vi "Live_Example.vi"() -> ()   [LabVIEW 2026]
doc: "This example demonstrates the image acquisition with one camera in ring buffer mode together with a live display of the latest images during record. After record is stopped, the images can be addressed by index.\nNote that this example will not be fail save, i.e. doesnt react on errors, just handles them forward to the end\n\nUsage:\nSelect your required image count, data format and the camera setup before you start the program.\nOnce started, the camera class will be initialized and images will be recorded and displayed automatically\nYou can stop the images by pressing stop record.\nAfter stopped, the image at the selected index will be read out\nTo finish the program click on quit application, this will force an exit of the camera class\nYou can change your required ROI after and also during the record."
uses:
  <instrlib>/PCO_SDK/File Group 0/vi.lib/Excelitas PCO GmbH/pco.labview/camera/Camera.lvclass
  <vilib>/picture/picture.llb/Draw 8-Bit Pixmap.vi
  <vilib>/picture/picture.llb/Draw True-Color Pixmap.vi
  <instrlib>/PCO_SDK/File Group 0/vi.lib/Excelitas PCO GmbH/pco.labview/pco.sdk/TimingControl/TimingControl.lvlib
panel:
  out "colormap(U8)":u32[](array[numeric])
  in  "Zoom [%]":i32(slide)=26 min=10 max=200 step=5 scale=10.0..200.0
  out "Image":picture
  out "Image(U16)":u16[][](graph)
  in  "Trigger":bool
  in  "data_format":T1(ring)=enum."Mono16"
  out "rawImage":u16[][](array[numeric])
  in  "Image Index":u32
  out "Recorded Images":u32
  in  "TriggerMode":T2(ring)
  in  "Quit":bool
  out "Error":errorcluster {"code" format="%x"}
  in  "Stop Record":bool
  out "Recording On":bool
  in  "roiY1":u64=2 min=1 max=1 step=1
  in  "roiX1":u64=2 min=1 max=1 step=1
  in  "roiY0":u64=1 max=1 step=1
  in  "roiX0":u64=1 max=1 step=1
  out "Image Height":u64
  out "Image Width":u64
  in  "dwImgCount":u32=10 caption="Required Number of Images" max=2397
  in  "Exposure Time [s]":dbl=0.010000000000000002 step=0.001
  # "This example demonstrates the image acquisition with one camera in ring buffer mode together with a live display of the latest images during record. After record is stopped, the images can be addressed by index.\nNote that this example will not be fail save, i.e. doesnt react on errors, just handles them forward to the end\n\nUsage:\nSelect your required image count, data format and the camera setup before you start the program.\nOnce started, the camera class will be initialized and images will be recorded and displayed automatically\nYou can stop the images by pressing stop record.\nAfter stopped, the image at the selected index will be read out\nTo finish the program click on quit application, this will force an exit of the camera class\nYou can change your required ROI after and also during the record."
  # "pco.labview"
  # "Camera Setup"
  # "Recording Control"
  # "Parameters for image readout"
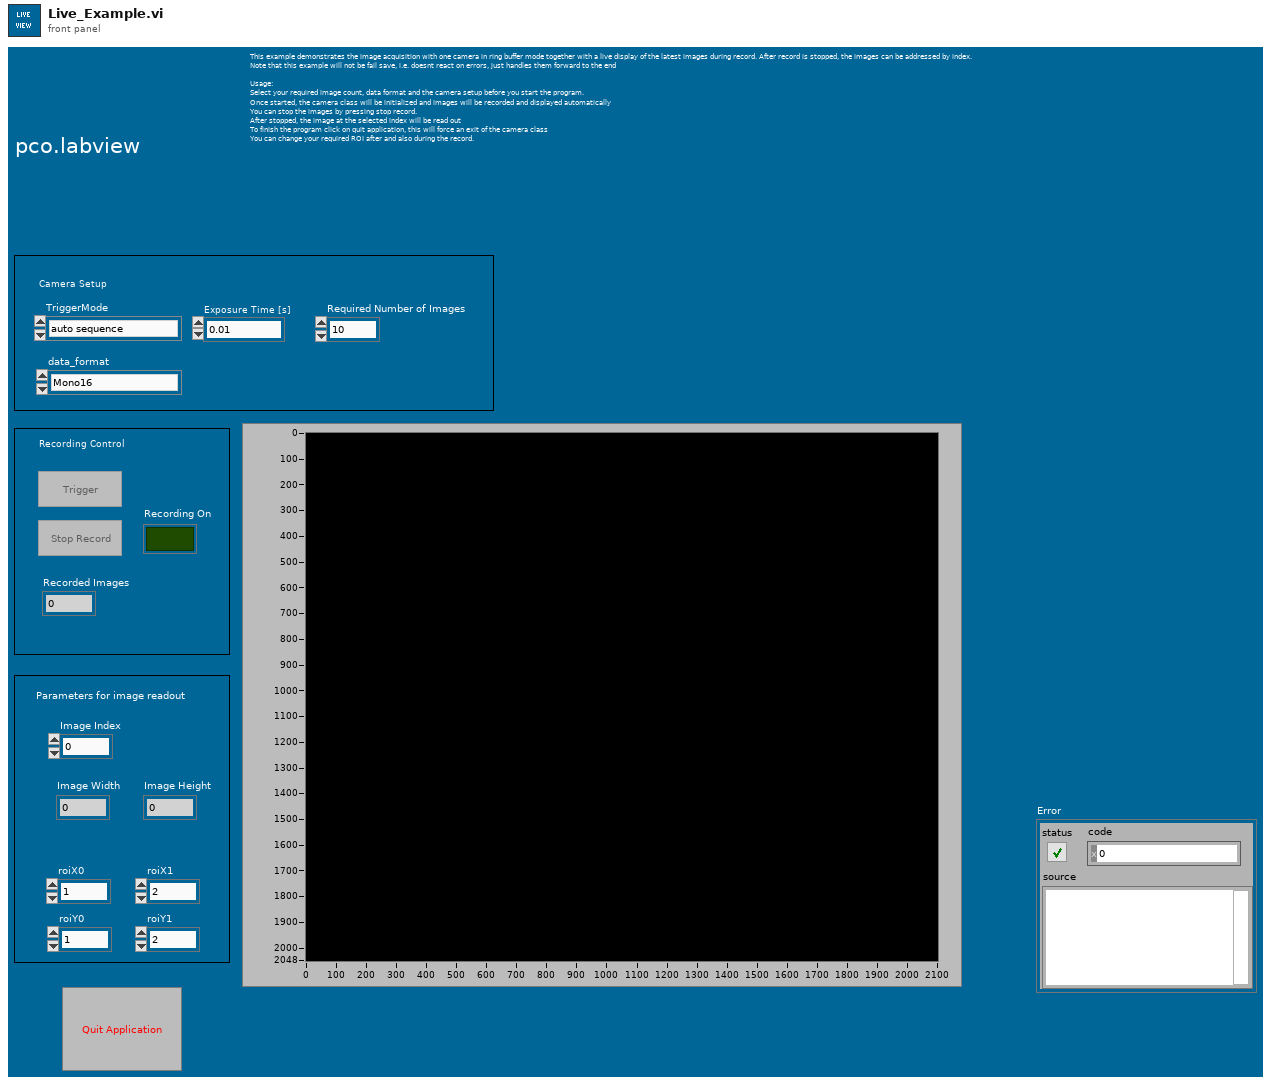
[diagram p1: front panel]
types:
  T1 = enum16{"Undefined", "Mono8", "Mono16", "BGRA8", "RGBA8", "BGRA16", "RGBA16", "CompressedMono8"}
  T2 = enum16{"auto sequence", "software trigger", "external exposure start", "external exposure control"}
  T3 = enum16{"sequence", "sequence non blocking", "ring buffer", "fifo", "sequence_dpcore", "sequence_non_blocking_dpcore", "ring_buffer_dpcore", "fifo_dpcore", "tif", "multitif", "pcoraw", "b16", "dicom", "multidicom", "camram_ring", "camram_segment"}
  T4 = enum8{"Enabled", "Disabled", "Disabled and Grayed Out"}
  T5 = cluster{"serial":u32, "type":u16, "sub_type":u16, "interface_type":u16, "bit_resolution":u16, "min_exposure_time_s":dbl, "max_exposure_time_s":dbl, "min_exposure_step_s":dbl, "min_delay_time_s":dbl, "max_delay_time_s":dbl, "min_delay_step_s":dbl, "min_width":u64, "min_height":u64, "max_width":u64, "max_height":u64, "roi_step_horz":u64, "roi_step_vert":u64, "roi_symmetric_horz":bool, "roi_symmetric_vert":bool, "has_timestamp_mode":bool, "has_timestamp_mode_ascii_only":bool, "pixelrate_vec":u32[], "has_acquire_mode":bool, "has_ext_acquire_mode":bool, "has_metadata_mode":bool, "has_ram":bool, "binning_horz_vec":u16[], "binning_vert_vec":u16[], "has_average_binning":bool, "pixel_format_vec":u32[], "has_trigger_mode_extexpctrl":bool}
  T6 = cluster{"wSignalNum":u16, "wEnabled":u16, "wType":u16, "wPolarity":u16, "wFilterSetting":u16, "wSelected":u16, "dwParameter":u32[], "dwSignalFunctionality":u32[]}
  T7 = typedef "Camera.lvclass/binning.ctl" = cluster{"vert":u16, "horz":u16, "mode":u16}
  T8 = cluster{"exposure_time_s":dbl, "delay_time_s":dbl, "roi":cluster{"x0":u64, "y0":u64, "x1":u64, "y1":u64}, "timestamp_mode":u16, "pixelrate":u32, "trigger_mode":u16, "acquire_mode":u16, "metadata_mode":u16, "noisefilter_mode":u16, "pixel_format":u32, "binning":T7, "auto_exposure":cluster{"region":u16, "min_exposure_s":dbl, "max_exposure_s":dbl}}
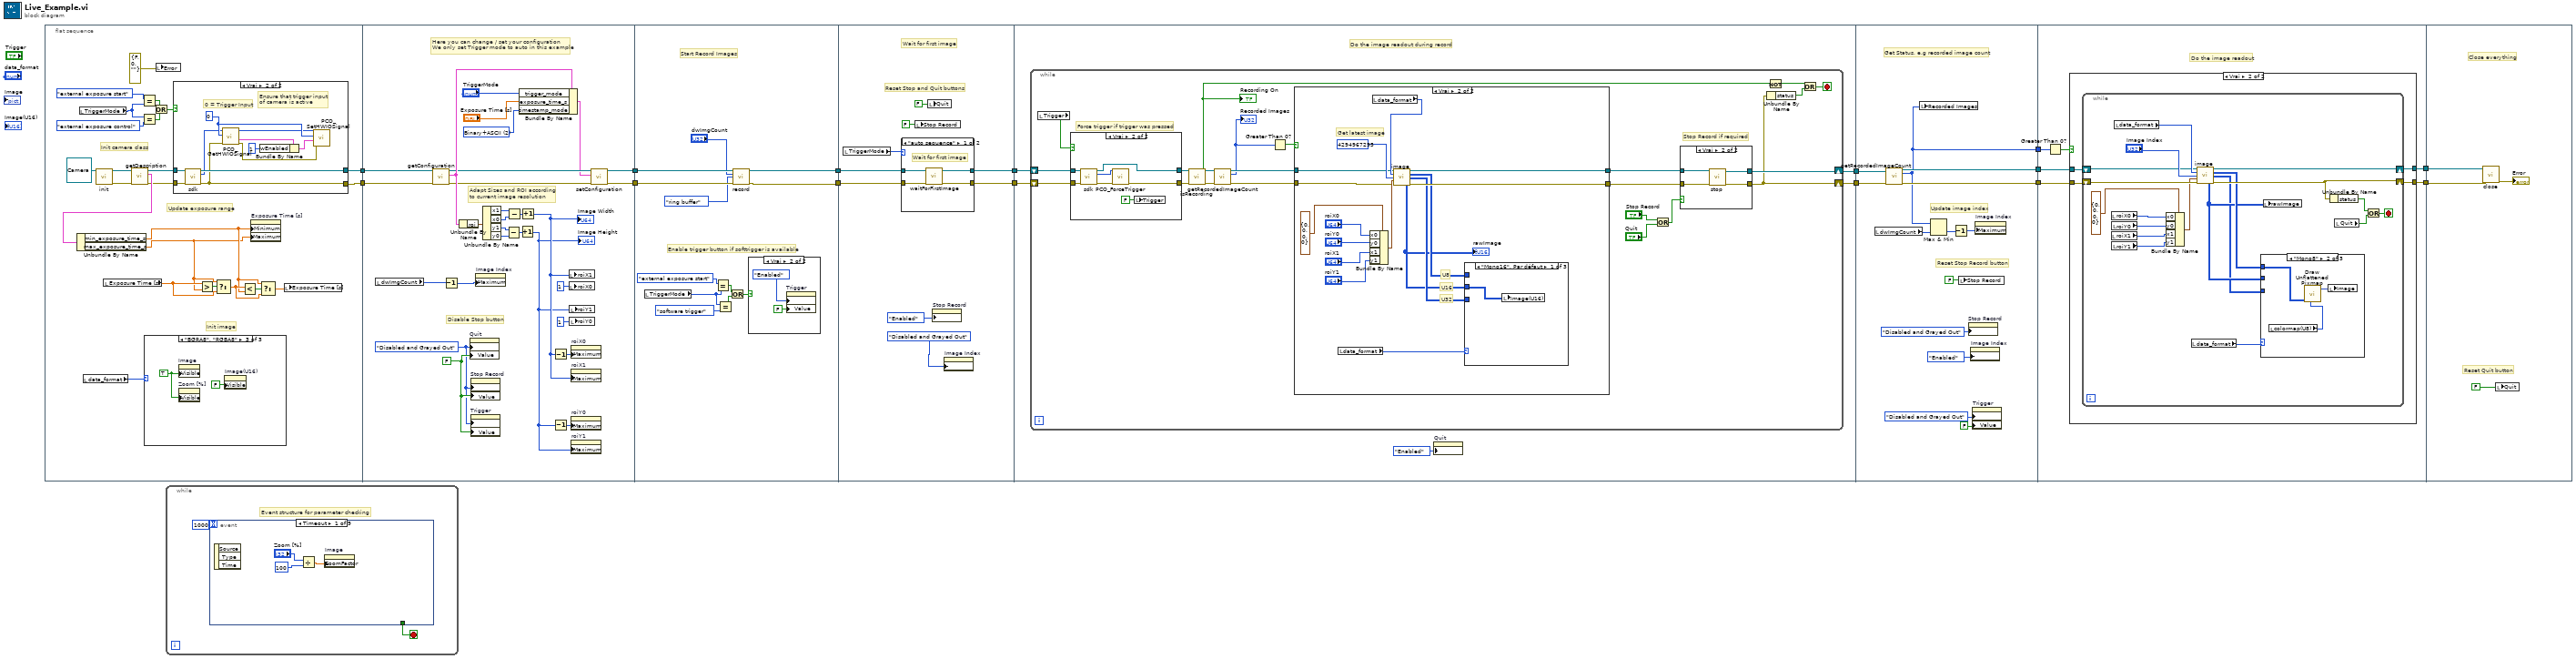
[diagram p0: block diagram]
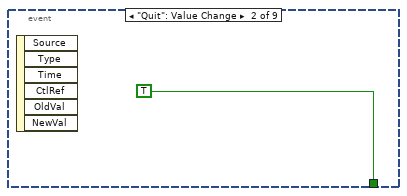
[diagram p2: hidden frame]
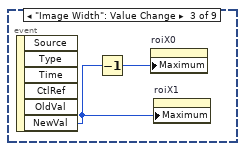
[diagram p3: hidden frame]
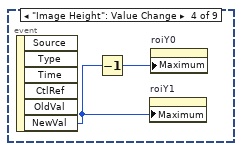
[diagram p4: hidden frame]
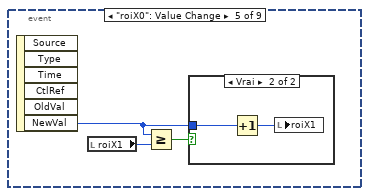
[diagram p5: hidden frame]
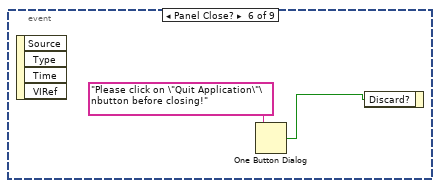
[diagram p7: hidden frame]
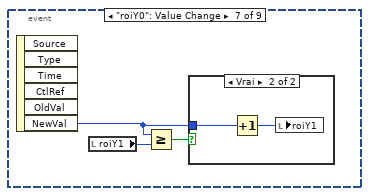
[diagram p8: hidden frame]
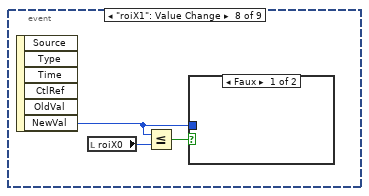
[diagram p10: hidden frame]
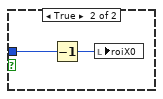
[diagram p11: hidden frame]
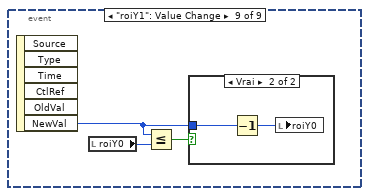
[diagram p12: hidden frame]
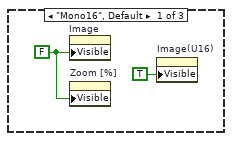
[diagram p15: hidden frame]
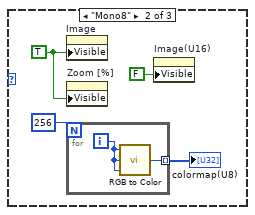
[diagram p16: hidden frame]
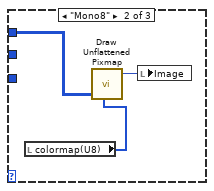
[diagram p20: hidden frame]
diagram:
  n1 = flat-sequence {
    tunnel: [w23] -> w7
    tunnel: [w16] -> w6
    tunnel: [w66] -> w15
    tunnel: [w70] -> w14
    tunnel: w7 -> [w65]
    tunnel: w6 -> [w64]
    tunnel: [w91] -> w9
    tunnel: [w92] -> w8
    tunnel: w14 -> [w101]
    tunnel: w15 -> [w100]
    tunnel: w9 -> [w108]
    tunnel: w8 -> [w109]
    tunnel: [w107] -> w13
    tunnel: [w105] -> w2
    tunnel: w13 -> [w123]
    tunnel: [w121] -> w12
    tunnel: [w120] -> w5
    tunnel: w2 -> [w119]
    tunnel: w12 -> [w194]
    tunnel: [w192] -> w11
    tunnel: w5 -> [w187]
    tunnel: [w186] -> w4
    tunnel: [w185] -> w1
    tunnel: w11 -> [w203]
    tunnel: [w202] -> w10
    tunnel: w4 -> [w201]
    tunnel: [w200] -> w3
    tunnel: w1 -> [w198]
    tunnel: w10 -> [w237]
    tunnel: w3 -> [w235]
    frame #0 {
      # "Init image"
      # "Init camera class"
      # "Update exposure range"
      n2 = local read "TriggerMode"() -> (w21:T2)
      n3 = local read "data_format"() -> (w26:T1)
      n4 = call-dynamic "init.vi"("Camera in"=refnum<class "Camera.lvclass"> refnum) -> ("Camera out"=w30:refnum<class "Camera.lvclass">, "error out"=w31:errorcluster)  [unwired: 8 in]
      n5 = local read "Exposure Time [s]"() -> (w37:dbl)
      n6 = call-dynamic "getDescription.vi"("error in (no error)"=w31, "Camera in"=w30) -> ("error out"=w25:errorcluster, "description"=w29:T5, "Camera out"=w24:refnum<class "Camera.lvclass">)  [unwired: 7 in]
      n7 = Unbundle By Name(w29) -> ("min_exposure_time_s"=w28:dbl, "max_exposure_time_s"=w27:dbl)
      n8 = Equal?(x=T2."external exposure start" ("TriggerMode"), y=w21) -> (x = y?=w19:bool)
      n9 = Equal?(x=w21, y=T2."external exposure control" ("TriggerMode")) -> (x = y?=w18:bool)
      n10 = case shown="\"BGRA8\", \"RGBA8\"" w26 {
        frame "Mono16", Default {
          w52 = FALSE ("Visible")
          n11 = property on="Image" class="Image"("Visible"=w52) -> ()  [unwired: 2 in, 2 out]
          n12 = property on="Zoom [%]" class="Gliss (strict)"("Visible"=w52) -> ()  [unwired: 2 in, 2 out]
          n13 = property on="Image(U16)" class="GraphInt (strict)"("Visible"=TRUE) -> ()  [unwired: 2 in, 2 out]
        }
        frame "Mono8" {
          w56 = TRUE ("Visible")
          n14 = property on="Image" class="Image"("Visible"=w56) -> ()  [unwired: 2 in, 2 out]
          n15 = property on="Zoom [%]" class="Gliss (strict)"("Visible"=w56) -> ()  [unwired: 2 in, 2 out]
          n16 = for {
            N: 256 -> [_]
            tunnel: [w58] -> w55 mode=indexing
            i -> [w59]
            n17 = call <vilib>:"RGB to Color.vi"("B"=w59, "G"=w59, "R"=w59) -> ("Color"=w58:u32)
          }
          "colormap(U8)" <- w55
          n18 = property on="Image(U16)" class="GraphInt (strict)"("Visible"=FALSE) -> ()  [unwired: 2 in, 2 out]
        }
        frame "BGRA8", "RGBA8" {
          w60 = TRUE ("Visible")
          n19 = property on="Image" class="Image"("Visible"=w60) -> ()  [unwired: 2 in, 2 out]
          n20 = property on="Zoom [%]" class="Gliss (strict)"("Visible"=w60) -> ()  [unwired: 2 in, 2 out]
          n21 = property on="Image(U16)" class="GraphInt (strict)"("Visible"=FALSE) -> ()  [unwired: 2 in, 2 out]
        }
      }
      n22 = Or(x=w19, y=w18) -> (x .or. y?=w17:bool)
      n23 = local write "Error"(errorcluster {"status"=FALSE, "code"=0, "source"=""} ("error IO")) -> ()
      n24 = case shown="Vrai" w17 {
        tunnel: w25 -> [w39 w45]
        tunnel: w24 -> [w40 w44]
        tunnel: [w40 w43] -> w23
        tunnel: [w39 w41] -> w16
        frame False {
        }
        frame True {
          w49 = u16 0 ("wSignalNum")
          # "0 = Trigger Input"
          # "Ensure that trigger input\nof camera is active"
          n25 = call-dynamic "sdk.vi"("Camera in"=w44, "error in (no error)"=w45) -> ("Camera out"=w43:refnum<class "Camera.lvclass">, "sdk"=w42:u64, "error out"=w41:errorcluster)  [unwired: 11 in]
          n26 = call <instrlib>:"PCO_GetHWIOSignal.vi"("error in (no error)"=w41, "wSignalNum"=w49, "ph"=w42) -> ("error out"=w47:errorcluster, "strSignal"=w51:T6, "ph out"=w46:u64)  [unwired: 5 in, 1 out]
          n27 = Bundle By Name(cluster=w51, "wEnabled"=u16 1) -> (w48:T6)
          n28 = call <instrlib>:"PCO_SetHWIOSignal.vi"("error in (no error)"=w47, "strSignal"=w48, "wSignalNum"=w49, "ph"=w46) -> ()  [unwired: 5 in, 3 out]
        }
      }
      n29 = Greater?(x=w37, y=w27) -> (0:w38:bool)
      n30 = Select(t=w27, s=w38, f=w37) -> (s? t:f=w35:dbl)
      n31 = Less?(x=w35, y=w28) -> (x < y?=w36:bool)
      n32 = property on="Exposure Time [s]" class="NumNb (strict)"("Minimum"=w28, "Maximum"=w27) -> ()  [unwired: 2 in, 2 out]
      n33 = Select(t=w28, s=w36, f=w35) -> (s? t:f=w34:dbl)
      n34 = local write "Exposure Time [s]"(w34) -> ()
    }
    frame #1 {
      w76 = u16 2 items=["OFF", "Binary", "Binary+ASCII", "ASCII"] ("wTimeStampMode")
      w63 = FALSE ("Stop")
      w62 = T4."Disabled and Grayed Out" ("Disabled")
      # "Disable Stop button"
      # "Adapt Sizes and ROI according\nto current image resolution"
      # "Here you can change / set your configuration\nWe only set Trigger mode to auto in this example"
      n35 = local read "dwImgCount"() -> (w77:u32)
      n36 = call-dynamic "getConfiguration.vi"("error in (no error)"=w64, "Camera in"=w65) -> ("error out"=w71:errorcluster, "configuration"=w82:T8, "Camera out"=w73:refnum<class "Camera.lvclass">)  [unwired: 7 in]
      n37 = Decrement(x=w77) -> (x-1=w67:u32)
      n38 = Unbundle By Name(w82) -> ("roi"=w83:cluster{"x0":u64, "y0":u64, "x1":u64, "y1":u64})
      n39 = property on="Quit" class="Bool (strict)"("DisabledEnum"=w62, "Value"=w63) -> ()  [unwired: 2 in, 2 out]
      n40 = property on="Stop Record" class="Bool (strict)"("DisabledEnum"=w62, "Value"=w63) -> ()  [unwired: 2 in, 2 out]
      n41 = property on="Trigger" class="Bool (strict)"("DisabledEnum"=w62, "Value"=w63) -> ()  [unwired: 2 in, 2 out]
      n42 = property on="Image Index" class="NumNb (strict)"("Maximum"=w67) -> ()  [unwired: 2 in, 2 out]
      n43 = Unbundle By Name(w83) -> ("x1"=w85:u64, "x0"=w84:u64, "y1"=w87:u64, "y0"=w86:u64)
      n44 = Subtract(x=w87, y=w86) -> (x-y=w89:u64)
      n45 = Subtract(x=w85, y=w84) -> (x-y=w88:u64)
      n46 = Bundle By Name(cluster=w82, "trigger_mode"="TriggerMode", "exposure_time_s"="Exposure Time [s]", "timestamp_mode"=w76) -> (w72:T8)
      n47 = Increment(x=w89) -> (x+1=w68:u64)
      "Image Height" <- w68
      n48 = Increment(x=w88) -> (x+1=w69:u64)
      "Image Width" <- w69
      n49 = Decrement(x=w69) -> (x-1=w80:u64)
      n50 = Decrement(x=w68) -> (x-1=w81:u64)
      n51 = local write "roiX1"(w69) -> ()
      n52 = local write "roiX0"(u64 1 ("roiY0")) -> ()
      n53 = local write "roiY1"(w68) -> ()
      n54 = local write "roiY0"(u64 1 ("roiY0")) -> ()
      n55 = property on="roiX0" class="NumNb (strict)"("Maximum"=w80) -> ()  [unwired: 2 in, 2 out]
      n56 = property on="roiX1" class="NumNb (strict)"("Maximum"=w69) -> ()  [unwired: 2 in, 2 out]
      n57 = property on="roiY0" class="NumNb (strict)"("Maximum"=w81) -> ()  [unwired: 2 in, 2 out]
      n58 = property on="roiY1" class="NumNb (strict)"("Maximum"=w68) -> ()  [unwired: 2 in, 2 out]
      n59 = call-dynamic "setConfiguration.vi"("error in (no error)"=w71, "configuration"=w72, "Camera in"=w73) -> ("error out"=w70:errorcluster, "Camera out"=w66:refnum<class "Camera.lvclass">)  [unwired: 7 in]
    }
    frame #2 {
      # "Enable trigger button if softtrigger is available"
      # "Start Record Images"
      n60 = local read "TriggerMode"() -> (w97:T2)
      n61 = Equal?(x=T2."external exposure start" ("TriggerMode"), y=w97) -> (x = y?=w94:bool)
      n62 = Equal?(x=w97, y=T2."software trigger" ("TriggerMode")) -> (x = y?=w93:bool)
      n63 = Or(x=w94, y=w93) -> (x .or. y?=w95:bool)
      n64 = call-dynamic "record.vi"("Camera in"=w100, "num_images"="dwImgCount", "record_mode"=T3."ring buffer", "error in (no error)"=w101) -> ("Camera out"=w92:refnum<class "Camera.lvclass">, "error out"=w91:errorcluster)  [unwired: 10 in]
      n65 = case shown="Vrai" w95 {
        frame False {
        }
        frame True {
          n66 = property on="Trigger" class="Bool (strict)"("DisabledEnum"=T4."Enabled" ("Disabled"), "Value"=FALSE ("Trigger")) -> ()  [unwired: 2 in, 2 out]
        }
      }
    }
    frame #3 {
      # "Wait for first image"
      # "Reset Stop and Quit buttons"
      n67 = local read "TriggerMode"() -> (w104:T2)
      n68 = case shown="\"auto sequence\"" w104 {
        tunnel: w109 -> [w116 w118]
        tunnel: w108 -> [w115 w117]
        tunnel: [w114 w117] -> w107
        tunnel: [w113 w118] -> w105
        frame "auto sequence" {
          # "Wait for first image"
          n69 = call-dynamic "waitForFirstImage.vi"("error in (no error)"=w115, "Camera in"=w116) -> ("error out"=w114:errorcluster, "Camera out"=w113:refnum<class "Camera.lvclass">)  [unwired: 8 in]
        }
        frame Default {
        }
      }
      n70 = local write "Stop Record"(FALSE ("Stop Record")) -> ()
      n71 = local write "Quit"(FALSE ("Stop")) -> ()
      n72 = property on="Stop Record" class="Bool (strict)"("DisabledEnum"=T4."Enabled" ("Disabled")) -> ()  [unwired: 2 in, 2 out]
      n73 = property on="Image Index" class="NumNb (strict)"("DisabledEnum"=T4."Disabled and Grayed Out" ("Disabled")) -> ()  [unwired: 2 in, 2 out]
    }
    frame #4 {
      # "Do the image readout during record"
      n74 = while {
        shift-right: [w126] -> w121
        shift-left: w123 -> [w130]
        shift-right: [w127] -> w120
        shift-left: w119 -> [w131]
        stop <- w142 stop-if-true
        # "Force trigger if trigger was pressed"
        # "Stop Record if required"
        n75 = local read "Trigger"() -> (w132:bool)
        n76 = case shown="Vrai" w132 {
          tunnel: w131 -> [w171 w176]
          tunnel: w130 -> [w170 w175]
          tunnel: [w171 w174] -> w129
          tunnel: [w170 w173] -> w128
          frame False {
          }
          frame True {
            n77 = call-dynamic "sdk.vi"("Camera in"=w176, "error in (no error)"=w175) -> ("Camera out"=w174:refnum<class "Camera.lvclass">, "sdk"=w177:u64, "error out"=w178:errorcluster)  [unwired: 11 in]
            n78 = call <instrlib>:"PCO_ForceTrigger.vi"("error in (no error)"=w178, "ph"=w177) -> ("error out"=w173:errorcluster)  [unwired: 6 in, 3 out]
            n79 = local write "Trigger"(FALSE ("Trigger")) -> ()
          }
        }
        n80 = call-dynamic "isRecording.vi"("Camera in"=w129, "error in (no error)"=w128) -> ("Camera out"=w137:refnum<class "Camera.lvclass">, "recording"=w140:bool, "error out"=w136:errorcluster)  [unwired: 11 in]
        "Recording On" <- w140
        n81 = call-dynamic "getRecordedImageCount.vi"("Camera in"=w137, "error in (no error)"=w136) -> ("Camera out"=w134:refnum<class "Camera.lvclass">, "recorded_image_count"=w124:u32, "error out"=w135:errorcluster)  [unwired: 11 in]
        "Recorded Images" <- w124
        n82 = Greater Than 0?(x=w124) -> (x > 0?=w125:bool)
        n83 = case shown="Vrai" w125 {
          tunnel: [w146 w158] -> w138
          tunnel: w135 -> [w146 w155]
          tunnel: w134 -> [w147 w149]
          tunnel: [w147 w148] -> w133
          frame False {
          }
          frame True {
            # "U32"
            # "U8"
            # "U16"
            # "Get latest image"
            n84 = local read "data_format"() -> (w150:T1)
            n85 = Bundle By Name(cluster=cluster{"x0":u64, "y0":u64, "x1":u64, "y1":u64} {"x0"=0, "y0"=0, "x1"=0, "y1"=0} ("roi"), "x0"="roiX0", "y0"="roiY0", "x1"="roiX1", "y1"="roiY1") -> (w159:cluster{"x0":u64, "y0":u64, "x1":u64, "y1":u64})
            n86 = local read "data_format"() -> (w154:T1)
            n87 = call-dynamic "image.vi"("Camera in"=w149, "data_format"=w154, "image_index"=u32 4294967295 ("dwImgIdx"), "roi"=w159, "error in (no error)"=w155) -> ("Camera out"=w148:refnum<class "Camera.lvclass">, "image (U8)"=w152:u8[][], "image (U32)"=w153:u32[][], "raw_image (U16)"=w151:u16[][], "error out"=w158:errorcluster)  [unwired: 2 in, 4 out]
            "rawImage" <- w151
            n88 = case shown="\"Mono16\", Par défaut" w150 {
              tunnel: w153 -> [_ _ w169]
              tunnel: w152 -> [_ w167 _]
              tunnel: w151 -> [w164 _ _]
              frame "Mono16", Default {
                n89 = local write "Image(U16)"(w164) -> ()
              }
              frame "Mono8" {
                n90 = local read "colormap(U8)"() -> (w166:u32[])
                n91 = call-poly <vilib>:"Draw Unflattened Pixmap.vi"("data"=w167, "color table"=w166) -> ("new picture"=w165:picture)  [unwired: 7 in]
                n92 = local write "Image"(w165) -> ()
              }
              frame "BGRA8", "RGBA8" {
                n93 = call-poly <vilib>:"Draw Unflattened Pixmap.vi"("data (RGB format)"=w169) -> ("new picture"=w168:picture)  [unwired: 8 in]
                n94 = local write "Image"(w168) -> ()
              }
            }
          }
        }
        n95 = Or(x="Stop Record", y="Quit") -> (x .or. y?=w143:bool)
        n96 = case shown="Vrai" w143 {
          tunnel: w138 -> [w180 w181]
          tunnel: [w179 w183] -> w127
          tunnel: [w180 w184] -> w126
          tunnel: w133 -> [w179 w182]
          frame False {
          }
          frame True {
            n97 = call-dynamic "stop.vi"("error in (no error)"=w181, "Camera in"=w182) -> ("error out"=w184:errorcluster, "Camera out"=w183:refnum<class "Camera.lvclass">)  [unwired: 8 in]
          }
        }
        n98 = Unbundle By Name(w126) -> ("status"=w141:bool)
        n99 = Not(x=w140) -> (.not. x?=w139:bool)
        n100 = Or(x=w139, y=w141) -> (x .or. y?=w142:bool)
      }
      n101 = property on="Quit" class="Bool (strict)"("DisabledEnum"=T4."Enabled" ("Disabled")) -> ()  [unwired: 2 in, 2 out]
    }
    frame #5 {
      # "Update image index"
      # "Reset Stop Record button"
      # "Get Status, e.g recorded image count"
      n102 = local read "dwImgCount"() -> (w193:u32)
      n103 = call-dynamic "getRecordedImageCount.vi"("Camera in"=w187, "error in (no error)"=w194) -> ("Camera out"=w186:refnum<class "Camera.lvclass">, "recorded_image_count"=w185:u32, "error out"=w192:errorcluster)  [unwired: 11 in]
      n104 = local write "Recorded Images"(w185) -> ()
      n105 = Max & Min(x=w185, y=w193) -> (min(x,y)=w195:u32)  [unwired: 1 out]
      n106 = Decrement(x=w195) -> (x-1=w190:u32)
      n107 = local write "Stop Record"(FALSE ("Stop Record")) -> ()
      n108 = property on="Stop Record" class="Bool (strict)"("DisabledEnum"=T4."Disabled and Grayed Out" ("Disabled")) -> ()  [unwired: 2 in, 2 out]
      n109 = property on="Image Index" class="NumNb (strict)"("DisabledEnum"=T4."Enabled" ("Disabled")) -> ()  [unwired: 2 in, 2 out]
      n110 = property on="Trigger" class="Bool (strict)"("DisabledEnum"=T4."Disabled and Grayed Out" ("Disabled"), "Value"=FALSE ("Trigger")) -> ()  [unwired: 2 in, 2 out]
      n111 = property on="Image Index" class="NumNb (strict)"("Maximum"=w190) -> ()  [unwired: 2 in, 2 out]
    }
    frame #6 {
      # "Do the image readout"
      n112 = Greater Than 0?(x=w198) -> (x > 0?=w199:bool)
      n113 = case shown="Vrai" w199 {
        tunnel: w203 -> [w204 w209]
        tunnel: [w204 w208] -> w202
        tunnel: w201 -> [w205 w207]
        tunnel: [w205 w206] -> w200
        frame False {
        }
        frame True {
          n114 = while {
            shift-right: [w220] -> w208
            shift-left: w209 -> [w228]
            shift-right: [w214] -> w206
            shift-left: w207 -> [w215]
            stop <- w222 stop-if-true
            n115 = local read "roiX0"() -> (w218:u64)
            n116 = local read "roiX1"() -> (w226:u64)
            n117 = local read "roiY0"() -> (w219:u64)
            n118 = local read "roiY1"() -> (w225:u64)
            n119 = local read "data_format"() -> (w216:T1)
            n120 = Bundle By Name(cluster=cluster{"x0":u64, "y0":u64, "x1":u64, "y1":u64} {"x0"=0, "y0"=0, "x1"=0, "y1"=0} ("roi"), "x0"=w218, "y0"=w219, "x1"=w226, "y1"=w225) -> (w227:cluster{"x0":u64, "y0":u64, "x1":u64, "y1":u64})
            n121 = local read "data_format"() -> (w213:T1)
            n122 = call-dynamic "image.vi"("Camera in"=w215, "data_format"=w216, "image_index"="Image Index", "roi"=w227, "error in (no error)"=w228) -> ("Camera out"=w214:refnum<class "Camera.lvclass">, "image (U8)"=w212:u8[][], "image (U32)"=w210:u32[][], "raw_image (U16)"=w211:u16[][], "error out"=w220:errorcluster)  [unwired: 2 in, 4 out]
            n123 = case shown="\"Mono8\"" w213 {
              tunnel: w210 -> [_ _ w234]
              tunnel: w212 -> [_ w232 _]
              tunnel: w211 -> [w229 _ _]
              frame "Mono16", Default {
                n124 = local write "Image(U16)"(w229) -> ()
              }
              frame "Mono8" {
                n125 = local read "colormap(U8)"() -> (w231:u32[])
                n126 = call-poly <vilib>:"Draw Unflattened Pixmap.vi"("data"=w232, "color table"=w231) -> ("new picture"=w230:picture)  [unwired: 7 in]
                n127 = local write "Image"(w230) -> ()
              }
              frame "BGRA8", "RGBA8" {
                n128 = call-poly <vilib>:"Draw Unflattened Pixmap.vi"("data (RGB format)"=w234) -> ("new picture"=w233:picture)  [unwired: 8 in]
                n129 = local write "Image"(w233) -> ()
              }
            }
            n130 = local write "rawImage"(w211) -> ()
            n131 = Unbundle By Name(w220) -> ("status"=w223:bool)
            n132 = local read "Quit"() -> (w224:bool)
            n133 = Or(x=w223, y=w224) -> (x .or. y?=w222:bool)
          }
        }
      }
    }
    frame #7 {
      # "Close everything"
      # "Reset Quit button"
      n134 = call-dynamic "close.vi"("error in (no error)"=w237, "Camera in"=w235) -> ("error out"=→"Error":errorcluster)  [unwired: 9 in]
      n135 = local write "Quit"(FALSE ("Stop Record")) -> ()
    }
  }
  n136 = while {
    stop <- w239 stop-if-true
    # "Event structure for parameter checking"
    n137 = event shown="[0] Timeout" {
      selector: _ -> [_ _ _ _ _ _ _ _ _]
      dyn-events: _ -> [_ _ _ _ _ _ _ _ _]
      timeout: 1000 -> [_ _ _ _ _ _ _ _ _]
      tunnel: [_ TRUE _ _ _ _ _ _ _] -> w239
      event Timeout {
        n138 = event-data() -> ()  [unwired: 1 in, 3 out]
        n139 = Divide(x="Zoom [%]", y=100 ("Zoom [%]")) -> (x/y=w242:dbl)
        n140 = property on="Image" class="Image"("ZoomFactor"=w242) -> ()  [unwired: 2 in, 2 out]
      }
      event "Quit": Value Change {
        n141 = event-data() -> ()  [unwired: 1 in, 6 out]
      }
      event "Image Width": Value Change {
        n142 = event-data() -> ("NewVal"=w245:u64)  [unwired: 1 in, 5 out]
        n143 = Decrement(x=w245) -> (x-1=w246:u64)
        n144 = property on="roiX0" class="NumNb (strict)"("Maximum"=w246) -> ()  [unwired: 2 in, 2 out]
        n145 = property on="roiX1" class="NumNb (strict)"("Maximum"=w245) -> ()  [unwired: 2 in, 2 out]
      }
      event "Image Height": Value Change {
        n146 = event-data() -> ("NewVal"=w247:u64)  [unwired: 1 in, 5 out]
        n147 = Decrement(x=w247) -> (x-1=w248:u64)
        n148 = property on="roiY1" class="NumNb (strict)"("Maximum"=w247) -> ()  [unwired: 2 in, 2 out]
        n149 = property on="roiY0" class="NumNb (strict)"("Maximum"=w248) -> ()  [unwired: 2 in, 2 out]
      }
      event "roiX0": Value Change {
        n150 = event-data() -> ("NewVal"=w249:u64)  [unwired: 1 in, 5 out]
        n151 = local read "roiX1"() -> (w251:u64)
        n152 = Greater Or Equal?(x=w249, y=w251) -> (x >= y?=w250:bool)
        n153 = case shown="Vrai" w250 {
          tunnel: w249 -> [_ w253]
          frame False {
          }
          frame True {
            n154 = Increment(x=w253) -> (x+1=w252:u64)
            n155 = local write "roiX1"(w252) -> ()
          }
        }
      }
      event Panel Close? {
        n156 = event-data() -> ()  [unwired: 1 in, 4 out]
        n157 = One Button Dialog(message="Please click on \"Quit Application\"\nbutton before closing!") -> (true=w254:bool)  [unwired: 1 in]
        n158 = event-data("Discard?"=w254) -> ()  [unwired: 1 in, 1 out]
      }
      event "roiY0": Value Change {
        n159 = event-data() -> ("NewVal"=w256:u64)  [unwired: 1 in, 5 out]
        n160 = local read "roiY1"() -> (w258:u64)
        n161 = Greater Or Equal?(x=w256, y=w258) -> (x >= y?=w257:bool)
        n162 = case shown="Vrai" w257 {
          tunnel: w256 -> [_ w260]
          frame False {
          }
          frame True {
            n163 = Increment(x=w260) -> (x+1=w259:u64)
            n164 = local write "roiY1"(w259) -> ()
          }
        }
      }
      event "roiX1": Value Change {
        n165 = event-data() -> ("NewVal"=w261:u64)  [unwired: 1 in, 5 out]
        n166 = local read "roiX0"() -> (w263:u64)
        n167 = Less Or Equal?(x=w261, y=w263) -> (x <= y?=w262:bool)
        n168 = case shown="Faux" w262 {
          tunnel: w261 -> [_ w265]
          frame False {
          }
          frame True {
            n169 = Decrement(x=w265) -> (x-1=w264:u64)
            n170 = local write "roiX0"(w264) -> ()
          }
        }
      }
      event "roiY1": Value Change {
        n171 = event-data() -> ("NewVal"=w266:u64)  [unwired: 1 in, 5 out]
        n172 = local read "roiY0"() -> (w268:u64)
        n173 = Less Or Equal?(x=w266, y=w268) -> (x <= y?=w267:bool)
        n174 = case shown="Vrai" w267 {
          tunnel: w266 -> [_ w270]
          frame False {
          }
          frame True {
            n175 = Decrement(x=w270) -> (x-1=w269:u64)
            n176 = local write "roiY0"(w269) -> ()
          }
        }
      }
    }
  }
